vi "zad4.vi"() -> ()   [LabVIEW 2017]
panel:
  in  "?":bool
  in  "stop":bool
  in  "?":bool
  in  "?":bool
  in  "?":bool
  in  "?":bool
  in  "?":bool
  in  "?":bool
  in  "?":bool
  in  "?":bool
  in  "?":bool
  out "Wynik":string
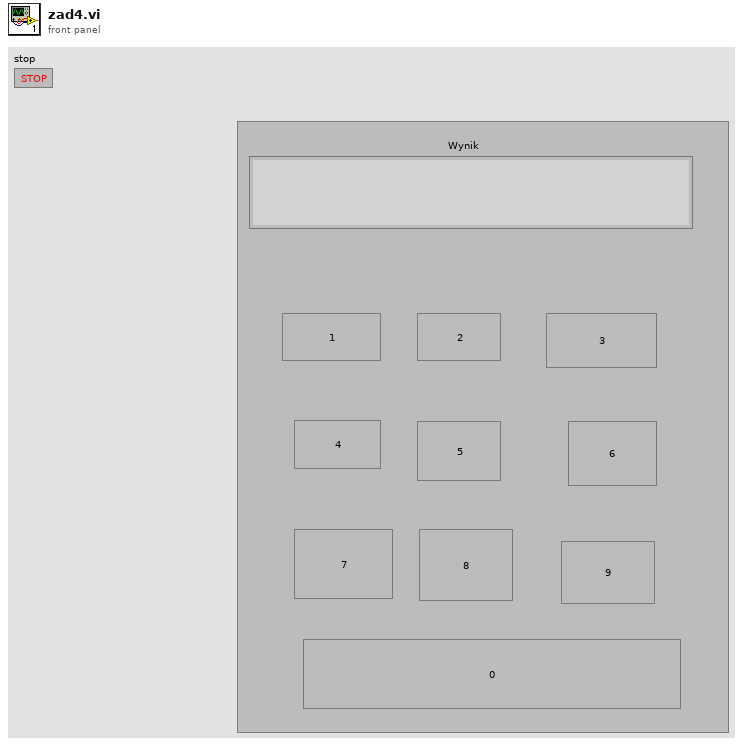
[diagram p1: front panel]
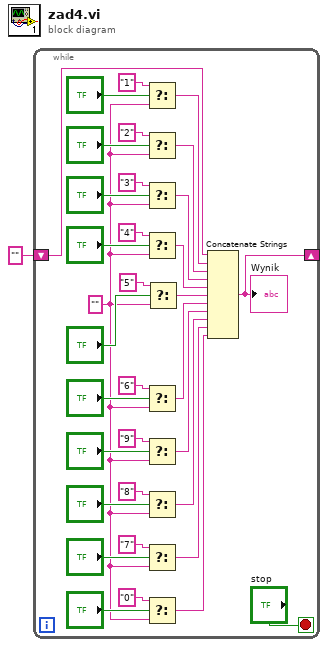
[diagram p0: block diagram]
diagram:
  n1 = while {
    shift-right: [w7] -> _
    shift-left: "" -> [w35]
    stop <- "stop" stop-if-true
    w4 = ""
    n2 = Select(t="1", s="?", f=w4) -> (s? t:f=w16:string)
    n3 = Select(t="2", s="?", f=w4) -> (s? t:f=w15:string)
    n4 = Select(t="3", s="?", f=w4) -> (s? t:f=w14:string)
    n5 = Select(t="4", s="?", f=w4) -> (s? t:f=w13:string)
    n6 = Select(t="6", s="?", f=w4) -> (s? t:f=w11:string)
    n7 = Select(t="9", s="?", f=w4) -> (s? t:f=w10:string)
    n8 = Select(t="8", s="?", f=w4) -> (s? t:f=w9:string)
    n9 = Select(t="7", s="?", f=w4) -> (s? t:f=w8:string)
    n10 = Select(t="0", s="?", f=w4) -> (s? t:f=w2:string)
    n11 = Select(t="5", s="?", f=w4) -> (s? t:f=w12:string)
    n12 = Concatenate Strings(w35, w16, w15, w14, w13, w12, w11, w10, w9, w8, w2) -> (w7:string)
    "Wynik" <- w7
  }
